vi "MdbPosEchoTableToCsv_topLevel.vi"() -> ()   [LabVIEW 2011]
uses:
  <vilib>/Utility/sysdir.llb/System Directory Type.ctl
  <vilib>/addons/database/Connection.llb/DB Tools Open Connec (String).vi
  <vilib>/addons/database/Connection.llb/DB Tools Open Connec (Path).vi
  <vilib>/addons/database/Connection.llb/Conn Get Properties.vi
  <vilib>/addons/database/_DB Variant To Data/Database Variant To Data.xnode
  <vilib>/addons/database/NI_Database_API.lvlib
panel:
  in  "Subcode":bool
  in  "Format":bool
  in  "ToTagFile":bool
  out "DbError":errorcluster[](array[cluster])
  out "FileRiteError":errorcluster[](array[cluster])
  in  "Footer":string
  in  "Header":string
  in  "Database Setup":bool
  out "NumberLeft":i32 caption="Number Left To Process"
  in  "Run":bool
  in  "Shutdown":bool
  out "Number of Files":i32 caption="Number of Files to Process"
  in  "pattern":string="*.mdb" caption="File Extention Type (*.type)"
  in  "scanMDB":path caption="Database Directory to scan (non-recursive)"
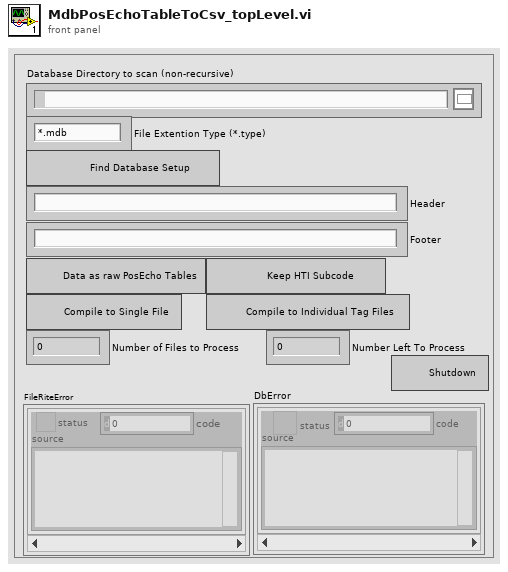
[diagram p1: front panel]
types:
  T1 = typedef "System Directory Type.ctl" = i32
  T2 = enum16{"open", "replace", "create", "open or create", "replace or create", "replace or create with confirmation"}
  T3 = typedef "NI_Database_API.lvlib/Conn ObjectReference.ctl" = refnum<k1>
  T4 = typedef "NI_Database_API.lvlib/Conn Properties.ctl" = cluster{"command timeout (s)":i32, "connection string":string, "default database":string, "provider":string}
  T5 = enum32{"invalid app kind", "Development System", "Run Time System", "Student Edition", "Embedded LabVIEW", "Evaluation", "Custom"}
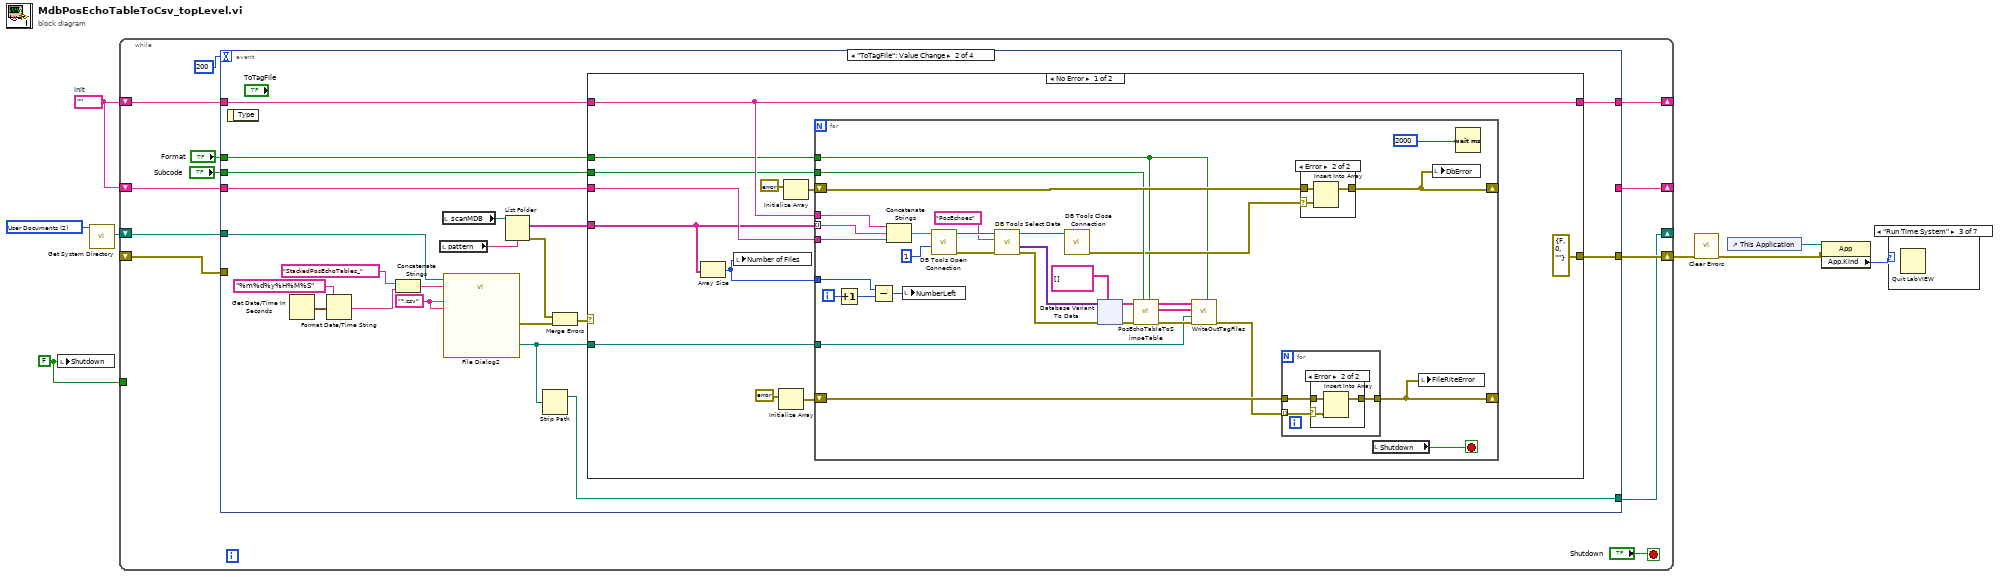
[diagram p0: block diagram]
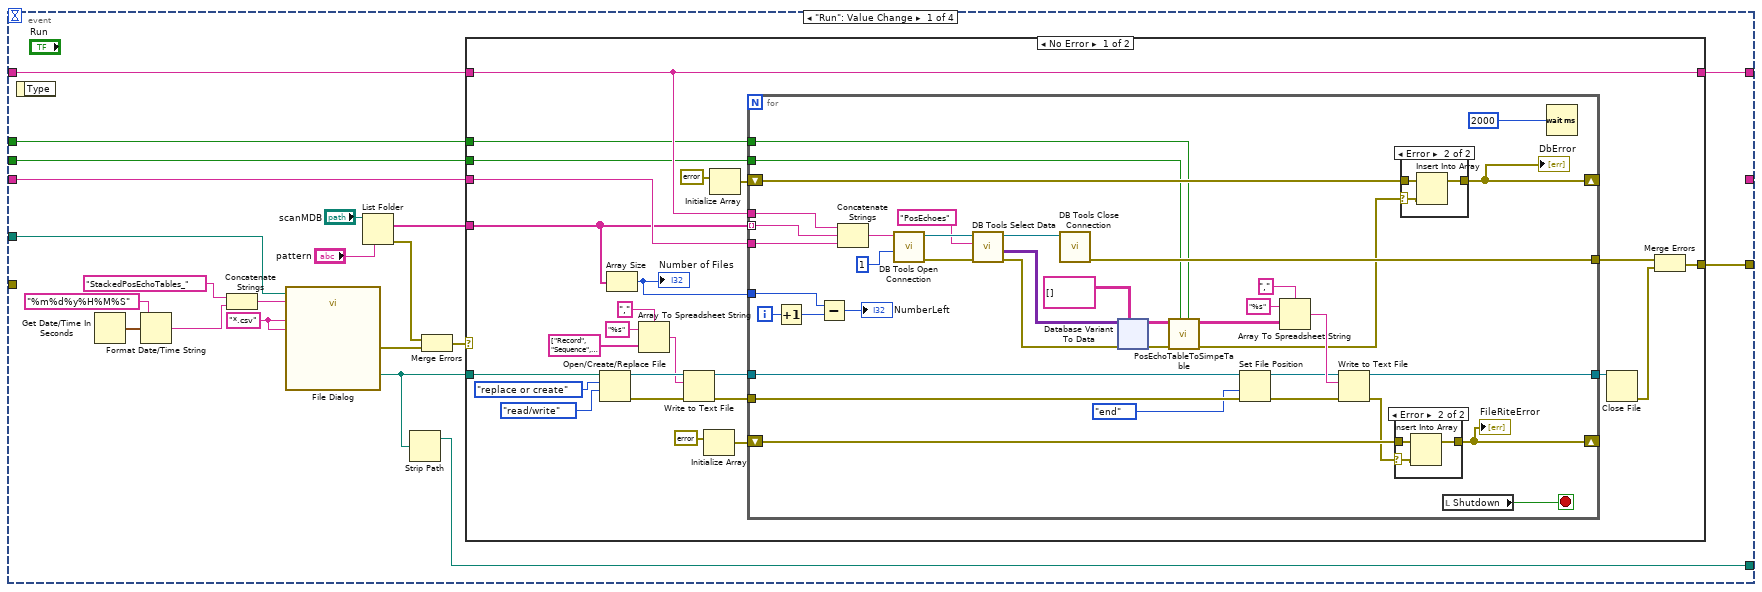
[diagram p8: hidden frame]
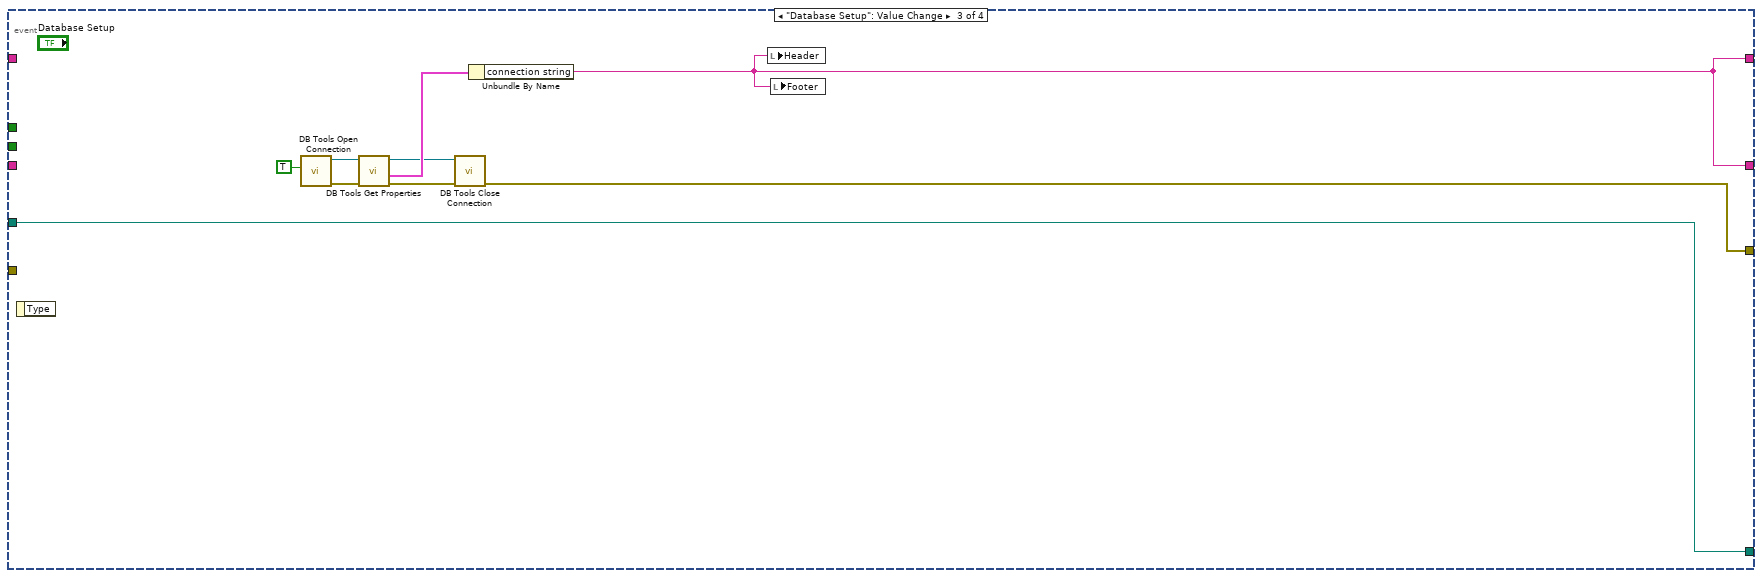
[diagram p15: hidden frame]
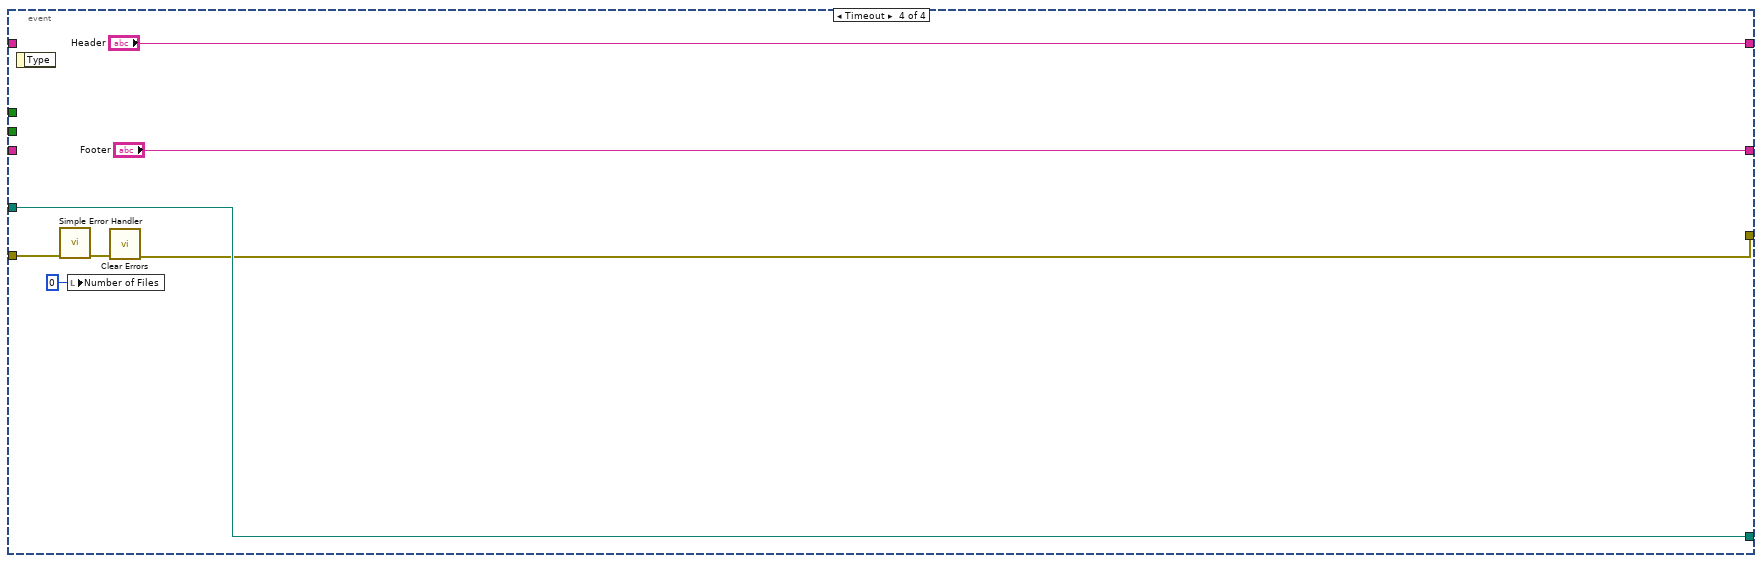
[diagram p16: hidden frame]
diagram:
  w1 = ""  # init
  w2 = FALSE ("Shutdown")
  w7 = T1 2 items=["User Home"=0, "User Desktop"=1, "User Documents"=2, "User Application Data"=3, "User Preferences"=4, "User Temporary"=5, "Public Documents"=6, "Public Application Data"=7, "Public Preferences"=8, "Public Cache"=13, "System Core Libraries"=9, "System Installed Libraries"=10, "Application Files"=11, "Boot Volume Root"=12] ("system directory type")
  n1 = local write "Shutdown"(w2) -> ()
  n2 = call <vilib>:"Get System Directory.vi"("system directory type"=w7) -> ("system directory"=w8:path)  [unwired: 10 in]
  n3 = while {
    shift-right: [w17] -> w4
    shift-left: _ -> [w16]
    shift-right: [w15] -> _
    shift-left: w1 -> [w14]
    shift-right: [w13] -> _
    shift-left: w8 -> [w20]
    tunnel: w2 -> [_]
    shift-right: [w11] -> _
    shift-left: w1 -> [w12]
    stop <- "Shutdown" stop-if-true
    n4 = event shown="[1] \"ToTagFile\": Value Change" {
      selector: _ -> [_ _ _ _]
      dyn-events: _ -> [_ _ _ _]
      timeout: 200 -> [_ _ _ _]
      tunnel: w20 -> [w41 w180 w284 w297]
      tunnel: [w30 w169 w283 w291] -> w17
      tunnel: w16 -> [_ _ _ w292]
      tunnel: [w34 w173 w282 "Header"] -> w15
      tunnel: w14 -> [w32 w171 _ _]
      tunnel: [w28 w168 w284 w297] -> w13
      tunnel: w12 -> [w31 w170 _ _]
      tunnel: [_ _ w282 "Footer"] -> w11
      tunnel: "Format" -> [w21 w162 _ _]
      tunnel: "Subcode" -> [w22 w161 _ _]
      event "Run": Value Change {
        w40 = "*.csv" ("pattern (all files)")
        n5 = event-data() -> ()  [unwired: 1 in, 1 out]
        n6 = Get Date/Time In Seconds() -> (seconds since 1Jan1904=w39:timestamp)
        n7 = Format Date/Time String(time format string (%c)="%m%d%y%H%M%S", seconds (now)=w39) -> (date/time string=w36:string)  [unwired: 1 in]
        n8 = Concatenate Strings("StackedPosEchoTables_" ("string"), w36) -> (w37:string)
        n9 = call "File Dialog"("start path"=w41, "default name"=w37, "pattern (all files)"=w40, "pattern label"=w40) -> ("selected path"=w29:path, "error out"=w33:errorcluster)  [unwired: 8 in, 2 out]
        n10 = List Folder(path="scanMDB", pattern="pattern") -> (filenames=w23:string[], error out=w24:errorcluster)  [unwired: 2 in, 2 out]
        n11 = Strip Path(path=w29) -> (stripped path=w28:path)  [unwired: 1 out]
        n12 = Merge Errors(w24, w33) -> (w25:errorcluster)
        n13 = case shown="No Error" w25 {
          selector: w25 -> [_ w159]
          tunnel: w29 -> [w66 _]
          tunnel: [w49 w159] -> w30
          tunnel: w32 -> [w54 w158]
          tunnel: [w54 w158] -> w34
          tunnel: w31 -> [w52 _]
          tunnel: w23 -> [w50 _]
          tunnel: w22 -> [w43 _]
          tunnel: w21 -> [w42 _]
          frame No Error {
            n14 = Open/Create/Replace File(file path (use dialog)=w66, operation (0:open)=T2."replace or create", access (0:read/write)=enum16{"read/write", "read-only", "write-only"}."read/write") -> (refnum out=w63:refnum<file>, error out=w62:errorcluster)  [unwired: 3 in, 1 out]
            n15 = Array Size(array=w50) -> (size(s)=w53:i32)
            "Number of Files" <- w53
            n16 = Array To Spreadsheet String(delimiter (Tab)=",", array=string[] ["Record", "Sequence", "TransmitLoc", "Period", "SubCode", "TrackType", "EchoTime", "PosX", "PosY", "PosZ", "ElevZ", "H1Record", "H2Record", "H3Record", "H4Record", "HD1", "HD2", "HD3", "HD4"] ("Array"), 3:"%s" ("format string")) -> (spreadsheet string=w58:string)
            n17 = Write to Text File(file (use dialog)=w63, text=w58, error in=w62) -> (refnum out=w61:refnum<file>, error out=w59:errorcluster)  [unwired: 1 in, 1 out]
            n18 = Initialize Array(errorcluster {"status"=FALSE, "code"=0, "source"=""} ("error constant")) -> (w47:errorcluster[])  [unwired: 1 in]
            n19 = Initialize Array(errorcluster {"status"=FALSE, "code"=0, "source"=""} ("error constant")) -> (w44:errorcluster[])  [unwired: 1 in]
            n20 = for {
              tunnel: w50 -> [w88] mode=indexing
              tunnel: w61 -> [w83]
              tunnel: [w100] -> w60
              tunnel: w59 -> [w81]
              tunnel: w54 -> [w95]
              tunnel: [w86] -> w51
              tunnel: w53 -> [w91]
              tunnel: w52 -> [w87]
              shift-right: [w76] -> _
              shift-left: w47 -> [w77]
              shift-right: [w73] -> _
              shift-left: w44 -> [w74]
              tunnel: w43 -> [w68]
              tunnel: w42 -> [w67]
              i -> [w92]
              stop <- w93 stop-if-true
              n21 = Increment(x=w92) -> (x+1=w90:i32)
              n22 = Subtract(x=w91, y=w90) -> (x-y=→"NumberLeft":i32)
              n23 = Concatenate Strings(w95, w88, w87) -> (w105:string)
              n24 = call-poly <vilib>:"DB Tools Open Connection.vi"("connection timeout (15)"=1, "connection information"=w105) -> ("error out"=w103:errorcluster, "connection reference"=w104:T3)  [unwired: 6 in]
              n25 = call <vilib>:"DB Tools Select Data.vi"("error in (no error)"=w103, "table"="PosEchoes", "connection reference"=w104) -> ("error out"=w78:errorcluster, "data"=w101:variant[][], "connection reference out"=w102:T3)  [unwired: 3 in]
              n26 = call <vilib>:"DB Tools Close Connection.vi"("connection reference"=w102) -> ("error out"=w86:errorcluster)  [unwired: 6 in]
              n27 = xnode "Database Variant To Data"("database variant"=w101, "error in"=w78, "type"=string[][] []) -> ("data"=w71:string[][], "error out"=w72:errorcluster)
              n28 = call "PosEchoTableToSimpeTable.vi"("Convert To Simple Table"=w67, "UpdateToRealSubcode(T=Real)"=w68, "error constant IN"=w72, "RawPosEchoTable"=w71) -> ("error out"=w69:errorcluster, "SimplePosTable"=w70:string[][])  [unwired: 5 in, 1 out]
              n29 = Set File Position(refnum=w83, from (0:start)=enum16{"start", "end", "current"}."end", error in=w81) -> (refnum out=w82:refnum<file>, error out=w80:errorcluster)  [unwired: 1 in]
              n30 = Array To Spreadsheet String(delimiter (Tab)=",", array=w70, 3:"%s" ("format string")) -> (spreadsheet string=w99:string)
              n31 = Write to Text File(file (use dialog)=w82, text=w99, error in=w80) -> (refnum out=w100:refnum<file>, error out=w75:errorcluster)  [unwired: 1 in, 1 out]
              n32 = case shown="Error" w75 {
                selector: w75 -> [_ w111]
                tunnel: w77 -> [w110 w113]
                tunnel: [w110 w112] -> w76
                frame No Error {
                }
                frame Error {
                  n33 = Insert Into Array(array=w113, new element=w111) -> (w112:errorcluster[])  [unwired: 1 in]
                }
              }
              "FileRiteError" <- w76
              n34 = case shown="Error" w69 {
                selector: w69 -> [_ w107]
                tunnel: w74 -> [w106 w109]
                tunnel: [w106 w108] -> w73
                frame No Error {
                }
                frame Error {
                  n35 = Insert Into Array(array=w109, new element=w107) -> (w108:errorcluster[])  [unwired: 1 in]
                }
              }
              "DbError" <- w73
              n36 = local read "Shutdown"() -> (w93:bool)
              n37 = Wait (ms)(milliseconds to wait=u32 2000) -> ()  [unwired: 1 out]
            }
            n38 = Close File(refnum=w60) -> (error out=w48:errorcluster)  [unwired: 1 in, 1 out]
            n39 = Merge Errors(w51, w48) -> (w49:errorcluster)
          }
          frame Error {
          }
        }
      }
      event "ToTagFile": Value Change {
        w179 = "*.csv" ("pattern (all files)")
        n40 = event-data() -> ()  [unwired: 1 in, 1 out]
        n41 = Get Date/Time In Seconds() -> (seconds since 1Jan1904=w178:timestamp)
        n42 = Format Date/Time String(time format string (%c)="%m%d%y%H%M%S", seconds (now)=w178) -> (date/time string=w175:string)  [unwired: 1 in]
        n43 = Concatenate Strings("StackedPosEchoTables_" ("string"), w175) -> (w176:string)
        n44 = local read "pattern"() -> (w163:string)
        n45 = local read "scanMDB"() -> (w164:path)
        n46 = call "File Dialog2"("start path"=w180, "default name"=w176, "pattern (all files)"=w179, "pattern label"=w179) -> ("selected path"=w160:path, "error out"=w172:errorcluster)  [unwired: 8 in, 2 out]
        n47 = List Folder(path=w164, pattern=w163) -> (filenames=w165:string[], error out=w166:errorcluster)  [unwired: 2 in, 2 out]
        n48 = Strip Path(path=w160) -> (stripped path=w168:path)  [unwired: 1 out]
        n49 = Merge Errors(w166, w172) -> (w167:errorcluster)
        n50 = case shown="No Error" w167 {
          selector: w167 -> [_ w281]
          tunnel: w160 -> [w182 _]
          tunnel: [errorcluster {"status"=FALSE, "code"=0, "source"=""} ("error IO") w281] -> w169
          tunnel: w171 -> [w192 w280]
          tunnel: [w192 w280] -> w173
          tunnel: w170 -> [w191 _]
          tunnel: w165 -> [w190 _]
          tunnel: w162 -> [w184 _]
          tunnel: w161 -> [w183 _]
          frame No Error {
            n51 = Array Size(array=w190) -> (size(s)=w185:i32)
            n52 = local write "Number of Files"(w185) -> ()
            n53 = Initialize Array(errorcluster {"status"=FALSE, "code"=0, "source"=""} ("error constant")) -> (w189:errorcluster[])  [unwired: 1 in]
            n54 = Initialize Array(errorcluster {"status"=FALSE, "code"=0, "source"=""} ("error constant")) -> (w186:errorcluster[])  [unwired: 1 in]
            n55 = for {
              tunnel: w190 -> [w212] mode=indexing
              tunnel: w192 -> [w217]
              tunnel: w185 -> [w214]
              tunnel: w191 -> [w211]
              shift-right: [w203] -> _
              shift-left: w189 -> [w207]
              shift-right: [w204] -> _
              shift-left: w186 -> [w206]
              tunnel: w184 -> [w193]
              tunnel: w183 -> [w200]
              tunnel: w182 -> [w196]
              i -> [w215]
              stop <- w216 stop-if-true
              n56 = Increment(x=w215) -> (x+1=w213:i32)
              n57 = Subtract(x=w214, y=w213) -> (x-y=w205:i32)
              n58 = Concatenate Strings(w217, w212, w211) -> (w224:string)
              n59 = local write "NumberLeft"(w205) -> ()
              n60 = call-poly <vilib>:"DB Tools Open Connection.vi"("connection timeout (15)"=1, "connection information"=w224) -> ("error out"=w222:errorcluster, "connection reference"=w223:T3)  [unwired: 6 in]
              n61 = call <vilib>:"DB Tools Select Data.vi"("error in (no error)"=w222, "table"="PosEchoes", "connection reference"=w223) -> ("error out"=w208:errorcluster, "data"=w220:variant[][], "connection reference out"=w221:T3)  [unwired: 3 in]
              n62 = call <vilib>:"DB Tools Close Connection.vi"("connection reference"=w221) -> ("error out"=w195:errorcluster)  [unwired: 6 in]
              n63 = xnode "Database Variant To Data"("database variant"=w220, "error in"=w208, "type"=string[][] []) -> ("data"=w201:string[][], "error out"=w202:errorcluster)
              n64 = call "PosEchoTableToSimpeTable.vi"("Convert To Simple Table"=w193, "UpdateToRealSubcode(T=Real)"=w200, "error constant IN"=w202, "RawPosEchoTable"=w201) -> ("error out"=w197:errorcluster, "TagList"=w198:string[], "SimplePosTable"=w199:string[][])  [unwired: 5 in]
              n65 = call "WriteOutTagFiles.vi"("SimpleDataset"=w193, "error IN"=w197, "file path (use dialog)"=w196, "TagList"=w198, "SimplePosTable"=w199) -> ("ErrorArray"=w194:errorcluster[])  [unwired: 6 in]
              n66 = for {
                tunnel: w207 -> [w227]
                tunnel: [w226] -> w203
                tunnel: w194 -> [w225] mode=indexing
                n67 = case shown="Error" w225 {
                  selector: w225 -> [_ w229]
                  tunnel: w227 -> [w228 w231]
                  tunnel: [w228 w230] -> w226
                  frame No Error {
                  }
                  frame Error {
                    n68 = Insert Into Array(array=w231, new element=w229) -> (w230:errorcluster[])  [unwired: 1 in]
                  }
                }
              }
              n69 = case shown="Error" w195 {
                selector: w195 -> [_ w233]
                tunnel: w206 -> [w232 w235]
                tunnel: [w232 w234] -> w204
                frame No Error {
                }
                frame Error {
                  n70 = Insert Into Array(array=w235, new element=w233) -> (w234:errorcluster[])  [unwired: 1 in]
                }
              }
              n71 = local read "Shutdown"() -> (w216:bool)
              n72 = local write "FileRiteError"(w203) -> ()
              n73 = local write "DbError"(w204) -> ()
              n74 = Wait (ms)(milliseconds to wait=u32 2000) -> ()  [unwired: 1 out]
            }
          }
          frame Error {
          }
        }
      }
      event "Database Setup": Value Change {
        n75 = event-data() -> ()  [unwired: 1 in, 1 out]
        n76 = call-poly <vilib>:"DB Tools Open Connection.vi"("prompt? (F)"=TRUE) -> ("error out"=w289:errorcluster, "connection reference"=w288:T3)  [unwired: 7 in]
        n77 = call-poly <vilib>:"DB Tools Get Properties.vi"("error in (no error)"=w289, "connection reference"=w288) -> ("error out"=w287:errorcluster, "connection properties"=w290:T4, "connection reference out"=w286:T3)  [unwired: 3 in]
        n78 = call <vilib>:"DB Tools Close Connection.vi"("error in (no error)"=w287, "connection reference"=w286) -> ("error out"=w283:errorcluster)  [unwired: 5 in]
        n79 = Unbundle By Name(w290) -> ("connection string"=w282:string)
        n80 = local write "Header"(w282) -> ()
        n81 = local write "Footer"(w282) -> ()
      }
      event Timeout {
        n82 = event-data() -> ()  [unwired: 1 in, 1 out]
        n83 = call <vilib>:"Simple Error Handler.vi"("error in (no error)"=w292) -> ("error out"=w293:errorcluster)  [unwired: 4 in, 4 out]
        n84 = local write "Number of Files"(0 ("Number of Files")) -> ()
        n85 = call <vilib>:"Clear Errors.vi"("error in (no error)"=w293) -> ("error out"=w291:errorcluster)  [unwired: 6 in]
      }
    }
  }
  n86 = call <vilib>:"Clear Errors.vi"("error in (no error)"=w4) -> ("error out"=w3:errorcluster)  [unwired: 6 in]
  n87 = control-ref of="This Application"() -> (w6:refnum<vi>)
  n88 = property class="App"(reference=w6, error in=w3) -> ("App.Kind"=w5:T5)  [unwired: 2 out]
  n89 = case shown="\"Run Time System\"" w5 {
    frame "invalid app kind", Default {
    }
    frame "Development System" {
    }
    frame "Run Time System" {
      n90 = Quit LabVIEW() -> ()  [unwired: 1 in]
    }
    frame "Student Edition" {
    }
    frame "Embedded LabVIEW" {
    }
    frame "Evaluation" {
    }
    frame "Custom" {
    }
  }
